vi "Default Instrument Setup.vi"(8 "error in (no error)":errorcluster, 11 "VISA resource name":refnum<visa-resource-name>) -> (0 "error out":errorcluster, 3 "VISA resource name out":refnum<visa-resource-name>)   [LabVIEW 2013, in "HadCon.lvlib"]
doc: "This Utility VI sends a default command string to the instrument whenever a new VISA session is opened, or the instrument is reset. Use this VI as a subVI for the Initialize and Reset VIs. Altering this VI could cause these two VIs to operate incorrectly."
uses:
  <instrlib>/HadCon/HadCon.lvlib
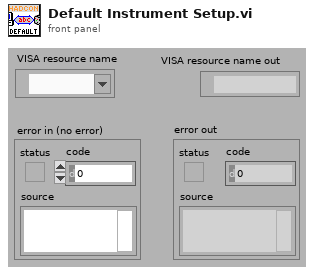
[diagram p1: front panel]
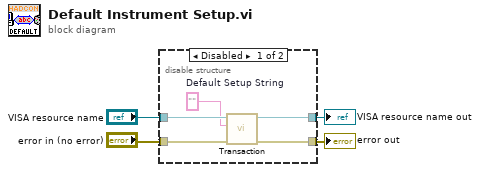
[diagram p0: block diagram]
diagram:
  n1 = disable-structure shown="Disabled" {
    disable-tunnel: "VISA resource name" -> [w9 w11]
    disable-tunnel: "error in (no error)" -> [w8 w10]
    disable-tunnel: [w7 w11] -> w2
    disable-tunnel: [w6 w10] -> w1
    frame Disabled {
      w5 = ""  # Default Setup String
      n2 = call <instrlib>:"Transaction.vi"("Error In"=w8, "Command"=w5, "VISA resource name"=w9) -> ("Error Out"=w6:errorcluster, "VISA resource name out"=w7:refnum<visa-resource-name>)  [unwired: 6 in, 1 out]
    }
    frame Enabled {
    }
  }
  "error out" <- w1
  "VISA resource name out" <- w2
